vi "Reset Font.vi"(6 "Variant in":variant, 7 "Shift Pressed?":bool, 8 "error in (no error)":errorcluster, 9 "Changed In":bool=TRUE, 10 "QD Combo Box Ref":refnum<vi>, 11 "QD Launch VI Ref":refnum<vi>) -> (0 "error out":errorcluster, 1 "Changed Out":bool=TRUE, 3 "QD Launch VI Ref":refnum<vi>, 4 "Variant out":variant)   [LabVIEW 2017]
doc: "Reset the font of the vi to the application font specified in LabVIEW.ini\n\nDefault Shortcut - [%]"
uses:
  <vilib>/regexp/Match Regular Expression.xnode
panel:
  in  "Undo Name":string="Reset Font"
  # "Specify the name of the Undo transaction"
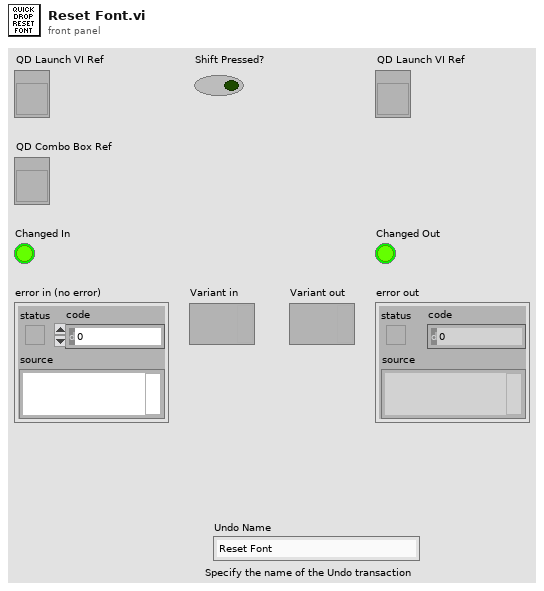
[diagram p1: front panel]
types:
  T1 = enum16{"open", "replace", "create", "open or create", "replace or create", "replace or create with confirmation"}
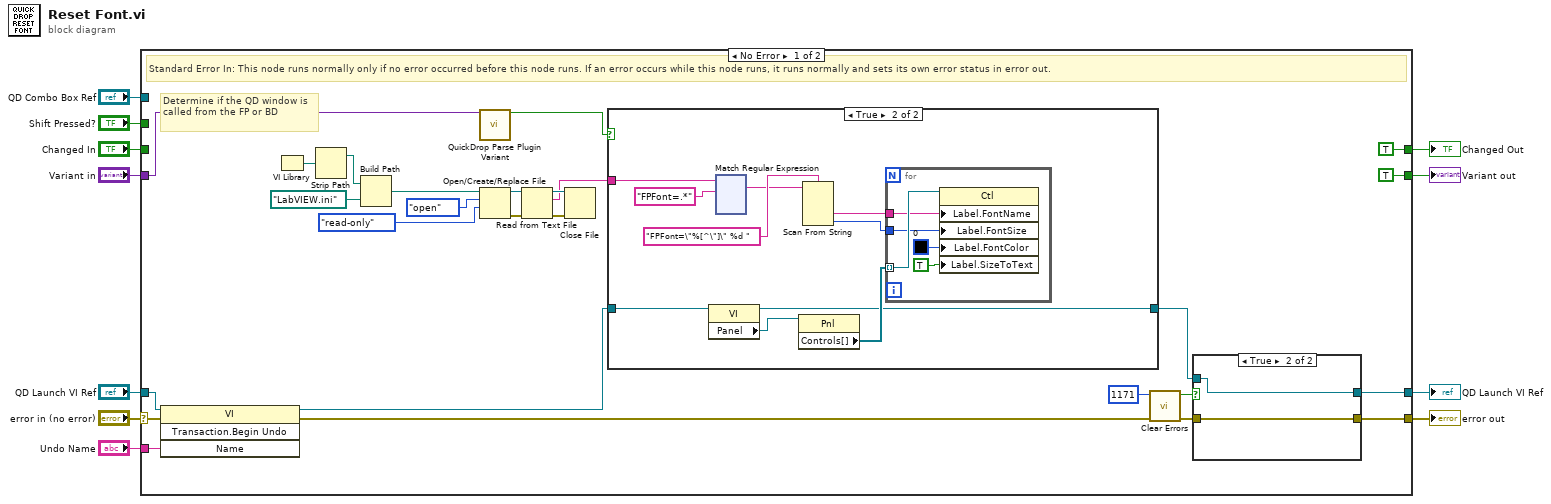
[diagram p0: block diagram]
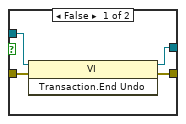
[diagram p2: hidden frame]
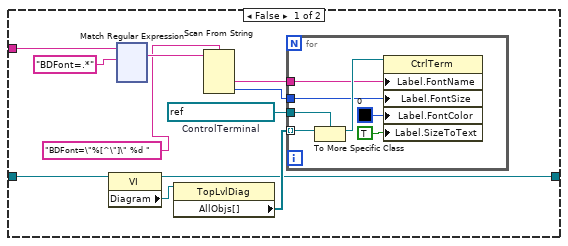
[diagram p3: hidden frame]
diagram:
  n1 = case shown="No Error" "error in (no error)" {
    selector: "error in (no error)" -> [w37 w307]
    tunnel: [w33 w307] -> w10
    tunnel: "QD Launch VI Ref" -> [w36 w305]
    tunnel: "Shift Pressed?" -> [_ _]
    tunnel: "QD Combo Box Ref" -> [_ _]
    tunnel: "Variant in" -> [w18 _]
    tunnel: "Undo Name" -> [w35 _]
    tunnel: [TRUE _] -> w5
    tunnel: [TRUE w306] -> w3
    tunnel: "Changed In" -> [_ w306]
    tunnel: [w16 w305] -> w1
    frame No Error {
      # "Determine if the QD window is called from the FP or BD"
      # "Standard Error In: This node runs normally only if no error occurred before this node runs. If an error occurs while this node runs, it runs normally and sets its own error status in error out."
      n2 = invoke class="VI" method="Transaction.Begin Undo"(reference=w36, error in=w37, "Name"=w35) -> (reference out=w20:refnum<vi>, error out=w15:errorcluster)  [unwired: 1 in, 2 out]
      n3 = VI Library() -> (path=w32:path)
      n4 = Strip Path(path=w32) -> (stripped path=w31:path)  [unwired: 1 out]
      n5 = Build Path(base path=w31, name or relative path=path "LabVIEW.ini") -> (appended path=w29:path)
      n6 = call <vilib>:"QuickDrop Parse Plugin Variant.vi"("QDKS Variant in"=w18) -> ("QD Launch VI Panel?"=w21:bool)  [unwired: 12 in, 2 out]
      n7 = Open/Create/Replace File(file path (use dialog)=w29, operation (0:open)=T1."open", access (0:read/write)=enum16{"read/write", "read-only", "write-only"}."read-only") -> (refnum out=w24:refnum<file>, error out=w26:errorcluster)  [unwired: 3 in, 1 out]
      n8 = Read from Text File(file (use dialog)=w24, error in=w26) -> (refnum out=w23:refnum<file>, text=w22:string, error out=w25:errorcluster)  [unwired: 2 in, 1 out]
      n9 = Close File(refnum=w23, error in=w25) -> ()  [unwired: 2 out]
      n10 = case shown="True" w21 {
        tunnel: w22 -> [w54 w183]
        tunnel: w20 -> [w46 w180]
        tunnel: [w44 w177] -> w19
        frame False {
          w49 = refnum<vi> refnum  # ControlTerminal
          n11 = property class="VI"(reference=w46) -> (reference out=w44:refnum<vi>, "Diagram"=w47:refnum<vi>)  [unwired: 1 in, 1 out]
          n12 = xnode "Match Regular Expression"("input string"=w54, "regular expression"="BDFont=.*") -> ("whole match"=w53:string)  [unwired: 4 in, 4 out]
          n13 = property class="TopLvlDiag"(reference=w47) -> ("AllObjs[]"=w45:refnum<vi>[])  [unwired: 1 in, 2 out]
          n14 = Scan From String(format string="BDFont=\"%[^\"]\" %d ", input string=w53) -> (output 1=w51:string, output 2=w50:i32)  [unwired: 4 in, 3 out]
          n15 = for {
            tunnel: w45 -> [w61] mode=indexing
            tunnel: w51 -> [w58]
            tunnel: w50 -> [w57]
            tunnel: w49 -> [w60]
            n16 = To More Specific Class(target class=w60, reference=w61) -> (specific class reference=w59:refnum<vi>)  [unwired: 1 in, 1 out]
            n17 = property class="CtrlTerm"(reference=w59, "Label.FontName"=w58, "Label.FontSize"=w57, "Label.FontColor"=u32 0, "Label.SizeToText"=TRUE ("Label.Size to Text?")) -> ()  [unwired: 1 in, 2 out]
          }
        }
        frame True {
          n18 = property class="VI"(reference=w180) -> (reference out=w177:refnum<vi>, "Panel"=w179:refnum<vi>)  [unwired: 1 in, 1 out]
          n19 = xnode "Match Regular Expression"("input string"=w183, "regular expression"="FPFont=.*") -> ("whole match"=w181:string)  [unwired: 4 in, 4 out]
          n20 = property class="Pnl"(reference=w179) -> ("Controls[]"=w178:refnum<vi>[])  [unwired: 1 in, 2 out]
          n21 = Scan From String(format string="FPFont=\"%[^\"]\" %d ", input string=w181) -> (output 1=w176:string, output 2=w184:i32)  [unwired: 4 in, 3 out]
          n22 = for {
            tunnel: w178 -> [w304] mode=indexing
            tunnel: w176 -> [w303]
            tunnel: w184 -> [w302]
            n23 = property class="Ctl"(reference=w304, "Label.FontName"=w303, "Label.FontSize"=w302, "Label.FontColor"=u32 0, "Label.SizeToText"=TRUE ("Label.Size to Text?")) -> ()  [unwired: 1 in, 2 out]
          }
        }
      }
      n24 = call <vilib>:"Clear Errors.vi"("error in (no error)"=w15, "specific error code to clear (0: all)"=1171) -> ("error out"=w14:errorcluster, "specific error cleared?"=w12:bool)  [unwired: 4 in]
      n25 = case shown="True" w12 {
        tunnel: [w41 w43] -> w33
        tunnel: w19 -> [w40 w42]
        tunnel: [w39 w42] -> w16
        tunnel: w14 -> [w38 w43]
        frame False {
          n26 = invoke class="VI" method="Transaction.End Undo"(reference=w40, error in=w38) -> (reference out=w39:refnum<vi>, error out=w41:errorcluster)  [unwired: 1 in, 1 out]
        }
        frame True {
        }
      }
    }
    frame Error {
      # "Standard Error In: If an error occurred before this node runs, the node passes the error in value to error out."
    }
  }
  "error out" <- w10
  "Variant out" <- w5
  "Changed Out" <- w3
  "QD Launch VI Ref" <- w1
